vi "Calc Dev.vi"(0 "Actual Table 1":string[][](array[string]), 1 "Actual Table 2":string[][](array[string]), 2 "Dev Table 1":string[][](array[string]), 3 "Dev Table 2":string[][](array[string]), 7 "Dev Table 1 Ref":refnum<vi>, 9 "Dev Table 2 Ref":refnum<vi>) -> (14 "Dev Table 1 OUT":string[][](array[string]), 15 "Dev Table 2 OUT":string[][](array[string]))   [LabVIEW 2013]
uses:
  <vilib>/Utility/miscctls.llb/LVRowAndColumnTypeDef.ctl
panel:
  out "appended array":string[][](array[string])
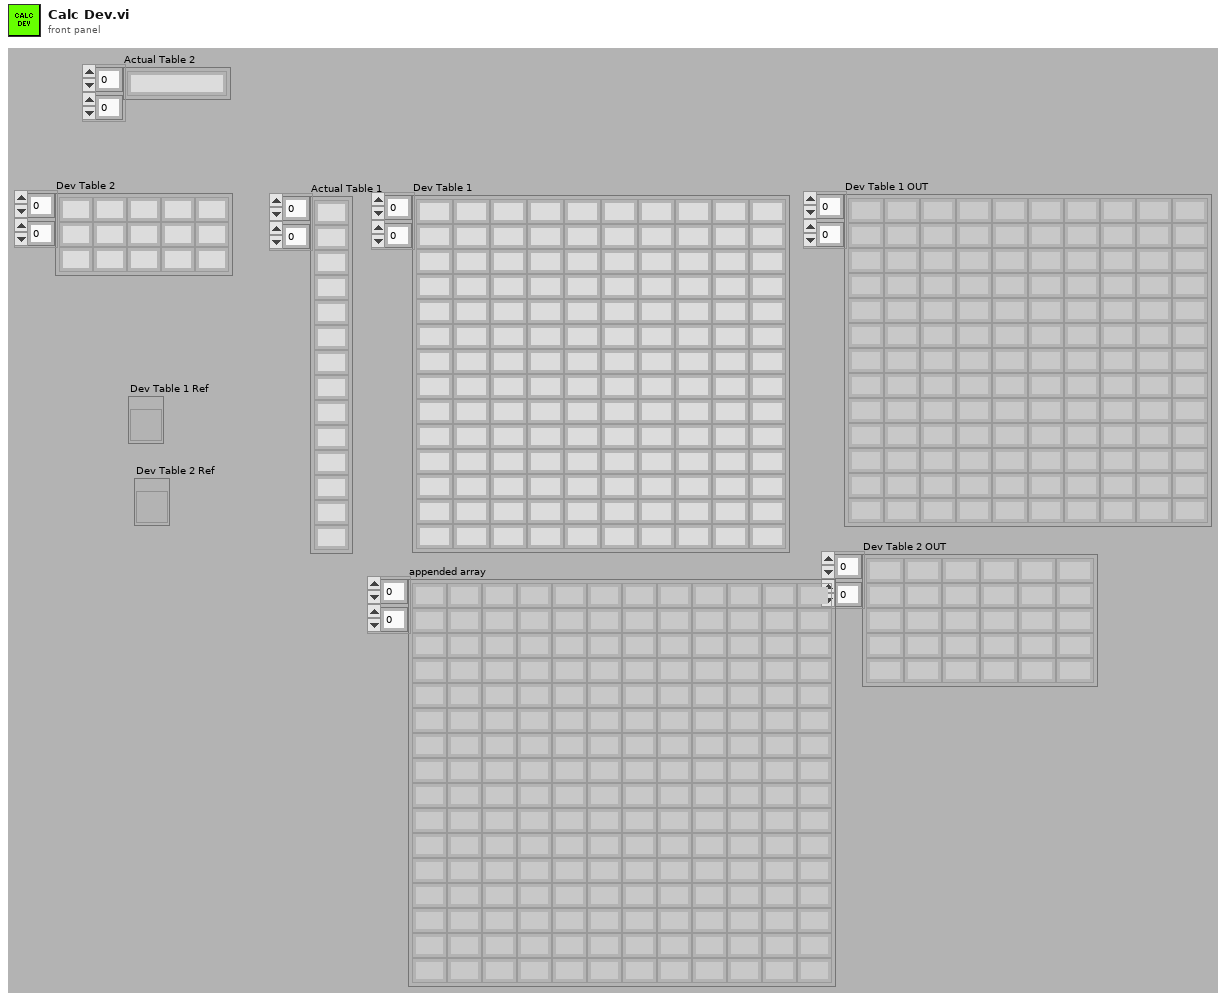
[diagram p1: front panel]
types:
  T1 = typedef "LVRowAndColumnTypeDef.ctl" = cluster{"Row":i32, "Column":i32}
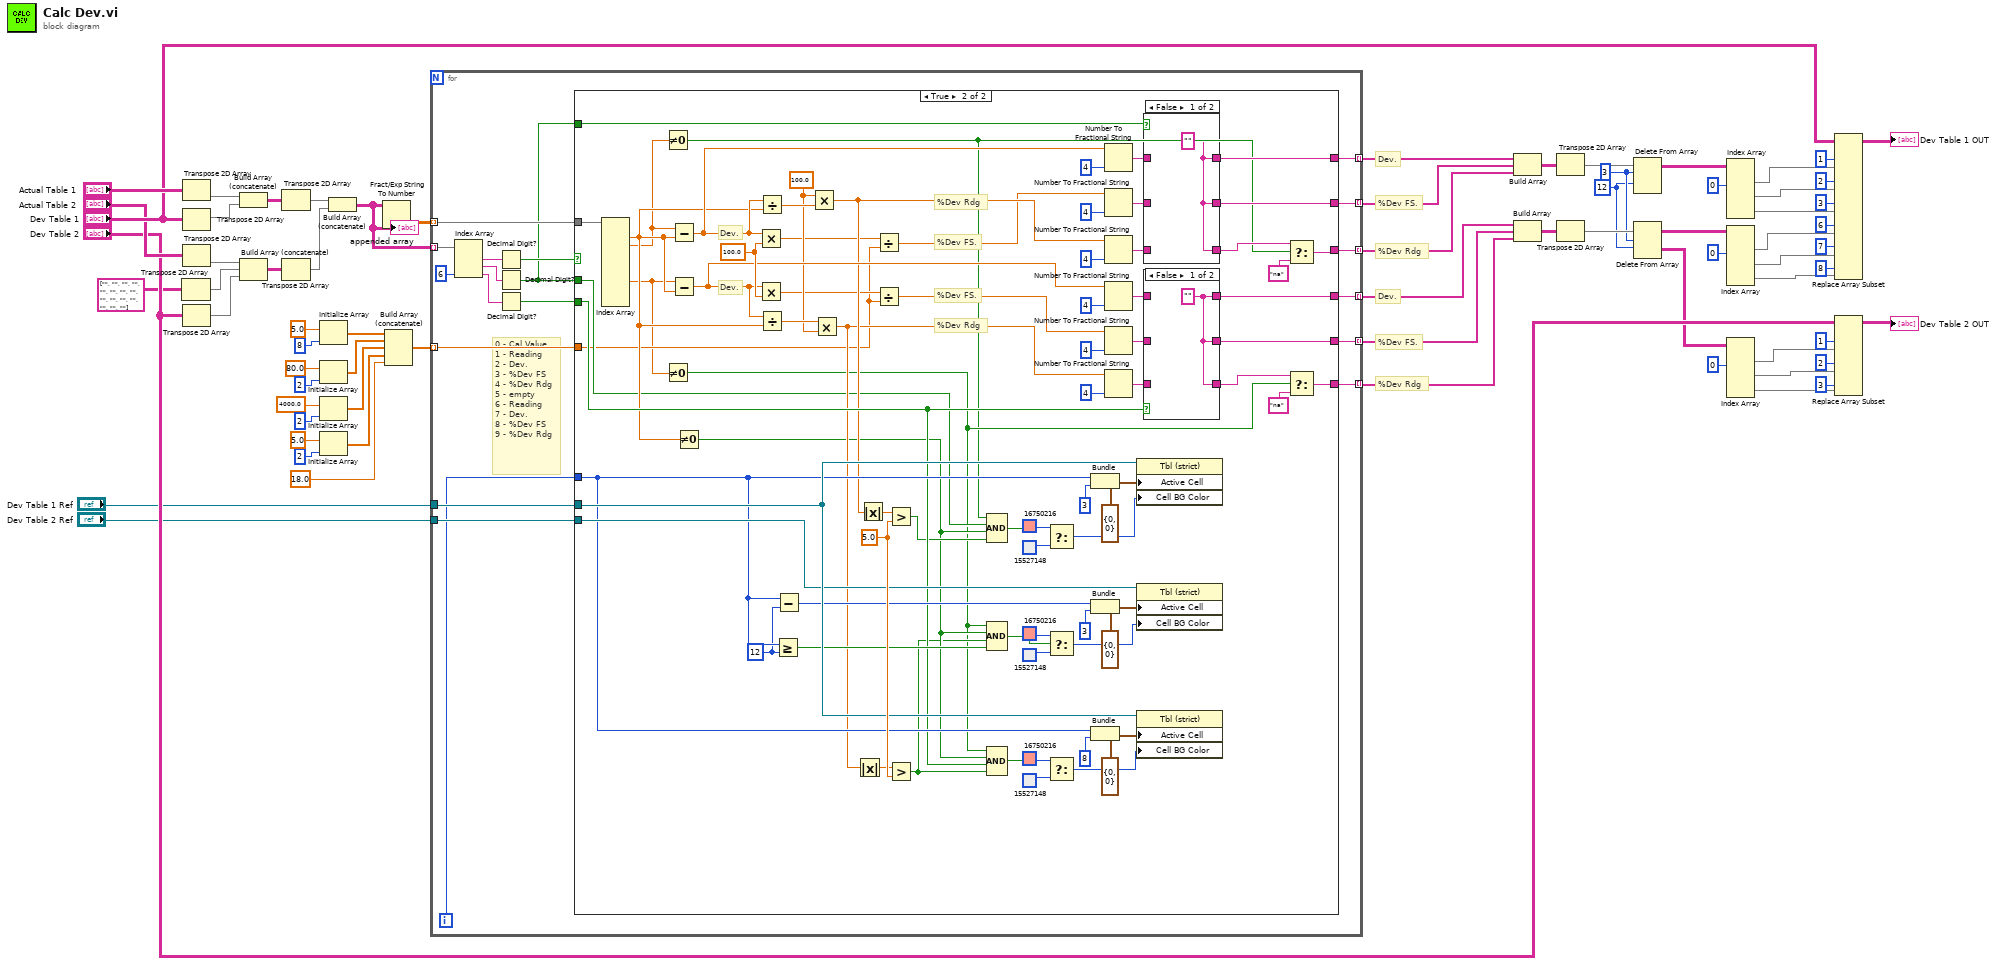
[diagram p0: block diagram]
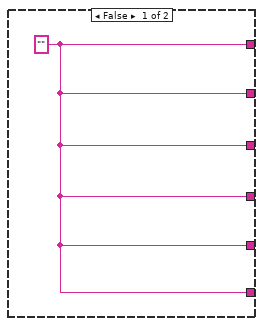
[diagram p2: hidden frame]
diagram:
  w59 = 3 ("length")
  w58 = 12 ("index (row)")
  # "%Dev Rdg"
  # "%Dev FS."
  # "Dev."
  # "%Dev Rdg"
  # "%Dev FS."
  # "Dev."
  n1 = Transpose 2D Array(2D array=string[][] [["", "", "", "", ""], ["", "", "", "", ""], ["", "", "", "", ""]] ("array")) -> (transposed array=w17:string[][])
  n2 = Transpose 2D Array(2D array="Actual Table 1") -> (transposed array=w30:string[][])
  n3 = Transpose 2D Array(2D array="Dev Table 1") -> (transposed array=w29:string[][])
  n4 = Transpose 2D Array(2D array="Actual Table 2") -> (transposed array=w28:string[][])
  n5 = Transpose 2D Array(2D array="Dev Table 2") -> (transposed array=w26:string[][])
  n6 = Build Array (concatenate)(w30, w29) -> (w31:string[][])
  n7 = Build Array (concatenate)(w28, w17, w26) -> (w27:string[][])
  n8 = Transpose 2D Array(2D array=w31) -> (transposed array=w23:string[][])
  n9 = Transpose 2D Array(2D array=w27) -> (transposed array=w22:string[][])
  n10 = Initialize Array(5.0, 8 ("dimension size")) -> (w6:dbl[])
  n11 = Initialize Array(80.0, 2 ("dimension size")) -> (w5:dbl[])
  n12 = Initialize Array(4000.0, 2 ("dimension size")) -> (w4:dbl[])
  n13 = Initialize Array(5.0, 2 ("dimension size")) -> (w3:dbl[])
  n14 = Build Array (concatenate)(w23, w22) -> (w21:string[][])
  "appended array" <- w21
  n15 = Fract/Exp String To Number(string=w21) -> (number=w70:dbl[][])  [unwired: 3 in, 1 out]
  n16 = Build Array (concatenate)(w6, w5, w4, w3, 18.0) -> (w1:dbl[])
  n17 = for {
    tunnel: w70 -> [w86] mode=indexing
    tunnel: w21 -> [w89] mode=indexing
    tunnel: [w85] -> w69 mode=indexing
    tunnel: [w84] -> w68 mode=indexing
    tunnel: [w83] -> w67 mode=indexing
    tunnel: [w82] -> w66 mode=indexing
    tunnel: [w81] -> w65 mode=indexing
    tunnel: [w80] -> w64 mode=indexing
    tunnel: "Dev Table 1 Ref" -> [w76]
    tunnel: "Dev Table 2 Ref" -> [w75]
    tunnel: w1 -> [w71] mode=indexing
    i -> [w74]
    # "0 - Cal Value\n1 - Reading\n2 - Dev.\n3 - %Dev FS\n4 - %Dev Rdg\n5 - empty\n6 - Reading\n7 - Dev.\n8 - %Dev FS\n9 - %Dev Rdg"
    n18 = Index Array(array=w89, index #3=6 ("index")) -> (element #1=w88:string, element #2=w87:string, element #3=w78:string)  [unwired: 2 in]
    n19 = Decimal Digit?(1:w88) -> (0:w73:bool)
    n20 = Decimal Digit?(1:w87) -> (0:w72:bool)
    n21 = Decimal Digit?(1:w78) -> (0:w77:bool)
    n22 = case shown="True" w73 {
      tunnel: w86 -> [_ w167]
      tunnel: [w90 w109] -> w85
      tunnel: [w90 w108] -> w84
      tunnel: [w90 w92] -> w83
      tunnel: [w90 w153] -> w82
      tunnel: [w90 w151] -> w81
      tunnel: [w90 w96] -> w80
      tunnel: w77 -> [_ w121]
      tunnel: w76 -> [_ w146]
      tunnel: w75 -> [_ w145]
      tunnel: w74 -> [_ w144]
      tunnel: w72 -> [_ w107]
      tunnel: w72 -> [_ w106]
      tunnel: w71 -> [_ w101]
      frame False {
        w90 = ""
      }
      frame True {
        w143 = 12 ("y")
        w149 = 5.0 ("y")
        w155 = 100.0 ("y")
        w166 = 100.0 ("y")
        # "%Dev Rdg"
        # "%Dev Rdg"
        # "%Dev FS."
        # "%Dev FS."
        # "Dev."
        # "Dev."
        n23 = Index Array(array=w167) -> (element #1=w115:dbl, element #2=w100:dbl, element #7=w99:dbl)  [unwired: 10 in, 7 out]
        n24 = Not Equal To 0?(x=w100) -> (x != 0?=w91:bool)
        n25 = Not Equal To 0?(x=w99) -> (x != 0?=w95:bool)
        n26 = Subtract(x=w100, y=w115) -> (x-y=w159:dbl)
        n27 = Subtract(x=w99, y=w115) -> (x-y=w157:dbl)
        n28 = Not Equal To 0?(x=w115) -> (x != 0?=w114:bool)
        n29 = Multiply(x=w159, y=w166) -> (x*y=w104:dbl)
        n30 = Multiply(x=w157, y=w166) -> (x*y=w103:dbl)
        n31 = Divide(x=w159, y=w115) -> (x/y=w158:dbl)
        n32 = Divide(x=w157, y=w115) -> (x/y=w156:dbl)
        n33 = Greater Or Equal?(x=w144, y=w143) -> (x >= y?=w122:bool)
        n34 = Subtract(x=w144, y=w143) -> (x-y=w142:i32)
        n35 = Multiply(x=w155, y=w158) -> (x*y=w119:dbl)
        n36 = Multiply(x=w156, y=w155) -> (x*y=w118:dbl)
        n37 = Absolute Value(x=w118) -> (abs(x)=w147:dbl)
        n38 = Absolute Value(x=w119) -> (abs(x)=w148:dbl)
        n39 = Divide(x=w104, y=w101) -> (x/y=w105:dbl)
        n40 = Divide(x=w103, y=w101) -> (x/y=w102:dbl)
        n41 = Greater?(x=w148, y=w149) -> (0:w117:bool)
        n42 = Greater?(x=w147, y=w149) -> (0:w113:bool)
        n43 = Compound Arithmetic op=AND(w91, w106, w114, w117) -> (w116:bool)
        n44 = Compound Arithmetic op=AND(w95, w114, w113, w122) -> (w123:bool)
        n45 = Compound Arithmetic op=AND(w95, w114, w121, w113) -> (w120:bool)
        n46 = Select(t=u32 16750216, s=w116, f=u32 15527148) -> (s? t:f=w130:u32)
        n47 = Select(t=u32 16750216, s=w123, f=u32 15527148) -> (s? t:f=w125:u32)
        n48 = Select(t=u32 16750216, s=w120, f=u32 15527148) -> (s? t:f=w124:u32)
        n49 = Bundle(cluster=T1 {"Row"=0, "Column"=0} ("Active Cell:Active Cell"), "Row"=w144, "Column"=3) -> (w140:T1)
        n50 = Bundle(cluster=T1 {"Row"=0, "Column"=0} ("Active Cell:Active Cell"), "Row"=w142, "Column"=3) -> (w137:T1)
        n51 = Bundle(cluster=T1 {"Row"=0, "Column"=0} ("Active Cell:Active Cell"), "Row"=w144, "Column"=8) -> (w134:T1)
        n52 = Number To Fractional String(number=w159, precision (6)=i16 4) -> (F-format string=w112:string)  [unwired: 2 in]
        n53 = Number To Fractional String(number=w105, precision (6)=i16 4) -> (F-format string=w111:string)  [unwired: 2 in]
        n54 = Number To Fractional String(number=w119, precision (6)=i16 4) -> (F-format string=w110:string)  [unwired: 2 in]
        n55 = Number To Fractional String(number=w157, precision (6)=i16 4) -> (F-format string=w154:string)  [unwired: 2 in]
        n56 = Number To Fractional String(number=w102, precision (6)=i16 4) -> (F-format string=w152:string)  [unwired: 2 in]
        n57 = Number To Fractional String(number=w118, precision (6)=i16 4) -> (F-format string=w150:string)  [unwired: 2 in]
        n58 = property on="Property Node" class="Tbl (strict)"(reference=w146, "Active Cell"=w140, "Cell BG Color"=w130) -> ()  [unwired: 1 in, 2 out]
        n59 = property on="Property Node" class="Tbl (strict)"(reference=w145, "Active Cell"=w137, "Cell BG Color"=w125) -> ()  [unwired: 1 in, 2 out]
        n60 = property on="Property Node" class="Tbl (strict)"(reference=w146, "Active Cell"=w134, "Cell BG Color"=w124) -> ()  [unwired: 1 in, 2 out]
        n61 = case shown="False" w107 {
          tunnel: [w168 w171] -> w109
          tunnel: w112 -> [_ w171]
          tunnel: w111 -> [_ w170]
          tunnel: [w168 w170] -> w108
          tunnel: w110 -> [_ w169]
          tunnel: [w168 w169] -> w93
          frame False {
            w168 = ""
          }
          frame True {
          }
        }
        n62 = case shown="False" w121 {
          tunnel: [w172 w175] -> w153
          tunnel: w154 -> [_ w175]
          tunnel: w152 -> [_ w174]
          tunnel: [w172 w174] -> w151
          tunnel: w150 -> [_ w173]
          tunnel: [w172 w173] -> w97
          frame False {
            w172 = ""
          }
          frame True {
          }
        }
        n63 = Select(t=w93, s=w91, f="na") -> (s? t:f=w92:string)
        n64 = Select(t=w97, s=w95, f="na") -> (s? t:f=w96:string)
      }
    }
  }
  n65 = Build Array(w69, w68, w67) -> (w63:string[][])
  n66 = Build Array(w66, w65, w64) -> (w62:string[][])
  n67 = Transpose 2D Array(2D array=w63) -> (transposed array=w61:string[][])
  n68 = Transpose 2D Array(2D array=w62) -> (transposed array=w60:string[][])
  n69 = Delete From Array(array=w61, length=w59, index (row)=w58) -> (array with subset deleted=w51:string[][])  [unwired: 1 in, 1 out]
  n70 = Delete From Array(array=w60, length=w59, index (row)=w58) -> (deleted portion=w15:string[][], array with subset deleted=w16:string[][])  [unwired: 1 in]
  n71 = Index Array(array=w51, index (col) #1=0 ("disabled index (col)")) -> (element #1=w49:string[], element #2=w48:string[], element #3=w47:string[])  [unwired: 5 in]
  n72 = Index Array(array=w16, index (col) #1=0 ("disabled index (col)")) -> (element #1=w45:string[], element #2=w44:string[], element #3=w43:string[])  [unwired: 5 in]
  n73 = Index Array(array=w15, index (col) #1=0 ("disabled index (col)")) -> (element #1=w37:string[], element #2=w36:string[], element #3=w35:string[])  [unwired: 5 in]
  n74 = Replace Array Subset(array="Dev Table 1", new element #1=w49, index (col) #1=1 ("disabled index (col)"), new element #2=w48, index (col) #2=2 ("index (col)"), new element #3=w47, index (col) #3=3 ("index (col)"), new element #4=w45, index (col) #4=6 ("index (col)"), new element #5=w44, index (col) #5=7 ("index (col)"), new element #6=w43, index (col) #6=8 ("index (col)")) -> (→"Dev Table 1 OUT":string[][])  [unwired: 6 in]
  n75 = Replace Array Subset(array="Dev Table 2", new element #1=w37, index (col) #1=1 ("disabled index (col)"), new element #2=w36, index (col) #2=2 ("index (col)"), new element #3=w35, index (col) #3=3 ("index (col)")) -> (→"Dev Table 2 OUT":string[][])  [unwired: 3 in]
